vi "Configure Trigger (RS232).vi"(0 "VISA resource name":refnum<visa-resource-name>, 5 "Trigger Source (1: Bus 1)":u16(ring)=1 items=["Bus 1"=1, "Bus 2"=2, "Bus 3"=3, "Bus 4"=4], 7 "Trigger Condition (0: RX Start)":u16(ring) items=["RX Start", "RX Data", "RX End Packet", "TX Start", "TX Data", "TX End Packet"], 9 "Data":T1={"Data Size (1)"=1, "Data Value (XXXXXXXX)"="XXXXXXXX"}, 11 "error in (no error)":errorcluster) -> (4 "VISA resource name out":refnum<visa-resource-name>, 15 "error out":errorcluster)   [LabVIEW 2009, in "Tektronix DPO MSO 2000 4000 Series.lvlib"]
doc: "Configures RS232 trigger settings for the oscilloscope."
uses:
  <instrlib>/Tektronix DPO MSO 2000 4000 Series/Tektronix DPO MSO 2000 4000 Series.lvlib
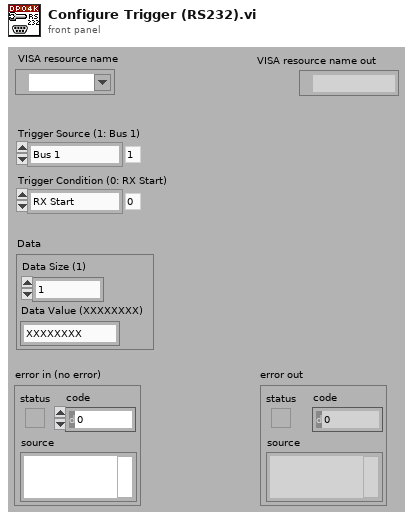
[diagram p1: front panel]
types:
  T1 = cluster{"Data Size (1)":i32, "Data Value (XXXXXXXX)":string}
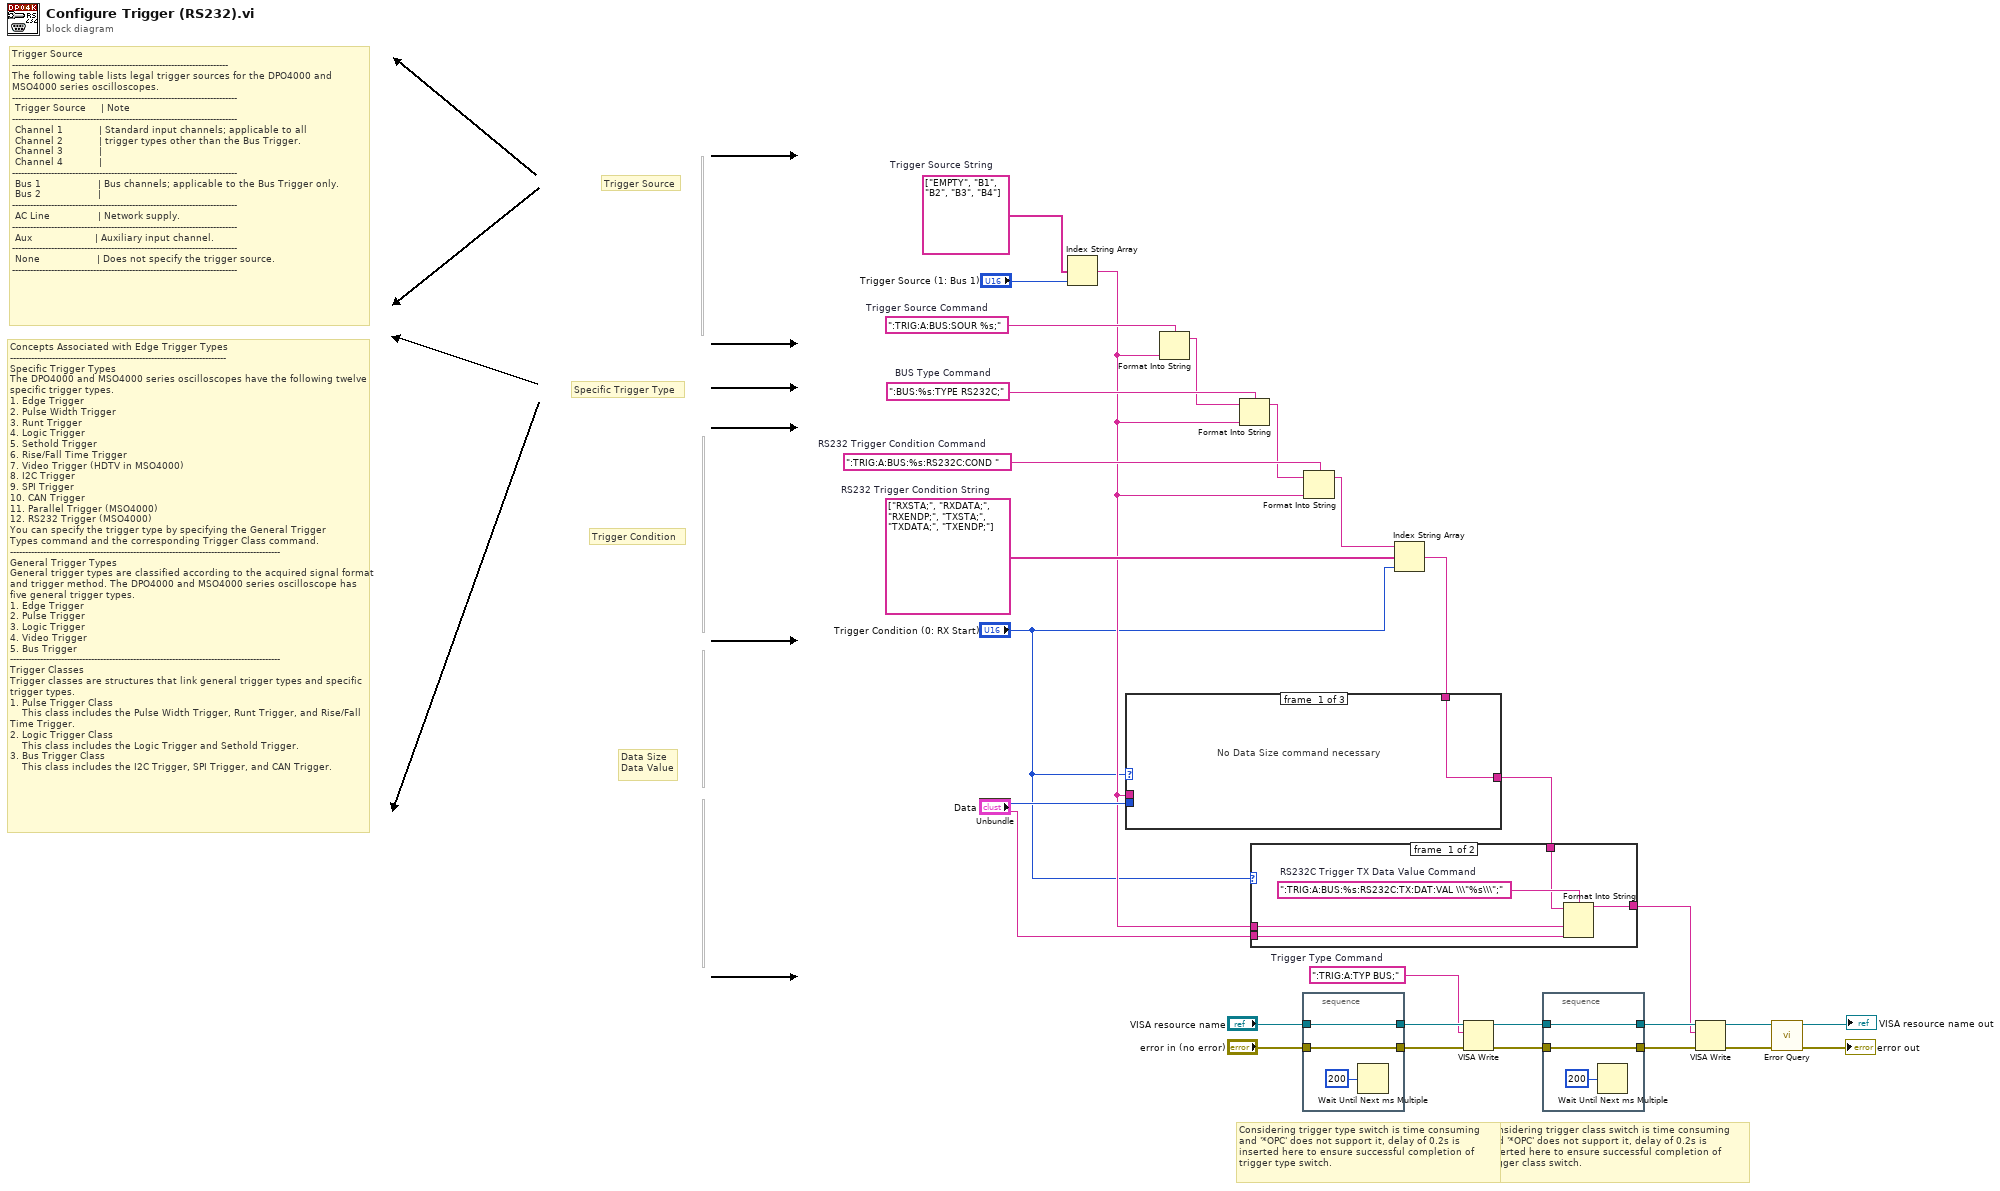
[diagram p0: block diagram]
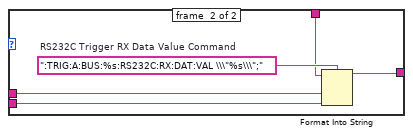
[diagram p2: hidden frame]
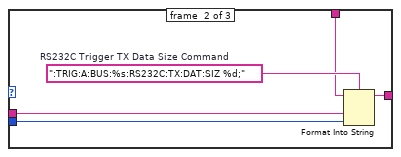
[diagram p3: hidden frame]
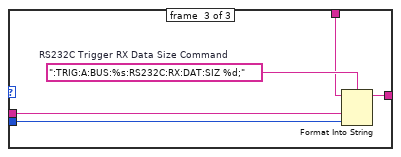
[diagram p4: hidden frame]
diagram:
  w22 = string[] ["EMPTY", "B1", "B2", "B3", "B4"]  # Trigger Source String
  w20 = ":TRIG:A:BUS:SOUR %s;"  # Trigger Source Command
  w24 = string[] ["RXSTA;", "RXDATA;", "RXENDP;", "TXSTA;", "TXDATA;", "TXENDP;"]  # RS232 Trigger Condition String
  w25 = ":TRIG:A:BUS:%s:RS232C:COND "  # RS232 Trigger Condition Command
  w21 = ":BUS:%s:TYPE RS232C;"  # BUS Type Command
  w28 = ":TRIG:A:TYP BUS;"  # Trigger Type Command
  # "Trigger Source\n------------------------------------------------------------------------\nThe following table lists legal trigger sources for the DPO4000 and MSO4000 series oscilloscopes.\n---------------------------------------------------------------------------\n Trigger Source     | Note                                                           \n---------------------------------------------------------------------------\n Channel 1            | Standard input channels; applicable to all      \n Channel 2            | trigger types other than the Bus Trigger.         \n Channel 3            |     \n Channel 4            |\n---------------------------------------------------------------------------\n Bus 1                   | Bus channels; applicable to the Bus Trigger only.\n Bus 2                   | \n---------------------------------------------------------------------------\n AC Line                | Network supply.\n---------------------------------------------------------------------------\n Aux                     | Auxiliary input channel.\n---------------------------------------------------------------------------\n None                   | Does not specify the trigger source.\n---------------------------------------------------------------------------"
  # "Concepts Associated with Edge Trigger Types\n------------------------------------------------------------------------\nSpecific Trigger Types\nThe DPO4000 and MSO4000 series oscilloscopes have the following twelve specific trigger types.\n1. Edge Trigger\n2. Pulse Width Trigger\n3. Runt Trigger\n4. Logic Trigger\n5. Sethold Trigger\n6. Rise/Fall Time Trigger\n7. Video Trigger (HDTV in MSO4000)\n8. I2C Trigger\n9. SPI Trigger\n10. CAN Trigger\n11. Parallel Trigger (MSO4000)\n12. RS232 Trigger (MSO4000)\nYou can specify the trigger type by specifying the General Trigger \nTypes command and the corresponding Trigger Class command.\n------------------------------------------------------------------------------------------\nGeneral Trigger Types \nGeneral trigger types are classified according to the acquired signal format and trigger method. The DPO4000 and MSO4000 series oscilloscope has five general trigger types.\n1. Edge Trigger\n2. Pulse Trigger\n3. Logic Trigger\n4. Video Trigger\n5. Bus Trigger\n------------------------------------------------------------------------------------------\nTrigger Classes\nTrigger classes are structures that link general trigger types and specific trigger types.\n1. Pulse Trigger Class\n    This class includes the Pulse Width Trigger, Runt Trigger, and Rise/Fall Time Trigger.\n2. Logic Trigger Class\n    This class includes the Logic Trigger and Sethold Trigger.\n3. Bus Trigger Class\n    This class includes the I2C Trigger, SPI Trigger, and CAN Trigger."
  # "Considering trigger class switch is time consuming\nand '*OPC' does not support it, delay of 0.2s is \ninserted here to ensure successful completion of\ntrigger class switch."
  # "Data Size\nData Value"
  # "Trigger Condition"
  # "Specific Trigger Type"
  # "Trigger Source"
  # "Considering trigger type switch is time consuming\nand '*OPC' does not support it, delay of 0.2s is \ninserted here to ensure successful completion of\ntrigger type switch."
  n1 = Unbundle("Data") -> ("Data Size (1)"=w8:i32, "Data Value (XXXXXXXX)"=w5:string)
  n2 = Index String Array(1:"Trigger Source (1: Bus 1)", 2:w22) -> (0:w6:string)  [unwired: 1 in]
  n3 = Format Into String(format string=w20, w6) -> (resulting string=w19:string)  [unwired: 2 in, 1 out]
  n4 = Format Into String(format string=w21, initial string=w19, w6) -> (resulting string=w18:string)  [unwired: 1 in, 1 out]
  n5 = stacked-sequence {
    tunnel: "VISA resource name" -> [w32]
    tunnel: [w32] -> w30
    tunnel: "error in (no error)" -> [w31]
    tunnel: [w31] -> w29
    frame #0 {
      n6 = Wait Until Next ms Multiple(millisecond multiple=u32 200) -> ()  [unwired: 1 out]
    }
  }
  n7 = Format Into String(format string=w25, initial string=w18, w6) -> (resulting string=w17:string)  [unwired: 1 in, 1 out]
  n8 = Index String Array(1:"Trigger Condition (0: RX Start)", 2:w24, 3:w17) -> (0:w7:string)
  n9 = case shown="0, Default" "Trigger Condition (0: RX Start)" {
    tunnel: [w34 w35 w40] -> w4
    tunnel: w6 -> [_ w36 w41]
    tunnel: w8 -> [_ w38 w43]
    tunnel: w7 -> [w34 w37 w42]
    frame #0 {
      # "No Data Size command necessary"
    }
    frame #1 {
      w39 = ":TRIG:A:BUS:%s:RS232C:TX:DAT:SIZ %d;"  # RS232C Trigger TX Data Size Command
      n10 = Format Into String(format string=w39, initial string=w37, w36, w38) -> (resulting string=w35:string)  [unwired: 1 in, 1 out]
    }
    frame #2 {
      w44 = ":TRIG:A:BUS:%s:RS232C:RX:DAT:SIZ %d;"  # RS232C Trigger RX Data Size Command
      n11 = Format Into String(format string=w44, initial string=w42, w41, w43) -> (resulting string=w40:string)  [unwired: 1 in, 1 out]
    }
  }
  n12 = case shown="0..2, Default" "Trigger Condition (0: RX Start)" {
    tunnel: [w48 w51] -> w3
    tunnel: w6 -> [w47 w54]
    tunnel: w5 -> [w46 w53]
    tunnel: w4 -> [w45 w50]
    frame #0 {
      w49 = ":TRIG:A:BUS:%s:RS232C:TX:DAT:VAL \\\"%s\\\";"  # RS232C Trigger TX Data Value Command
      n13 = Format Into String(format string=w49, initial string=w45, w47, w46) -> (resulting string=w48:string)  [unwired: 1 in, 1 out]
    }
    frame #1 {
      w52 = ":TRIG:A:BUS:%s:RS232C:RX:DAT:VAL \\\"%s\\\";"  # RS232C Trigger RX Data Value Command
      n14 = Format Into String(format string=w52, initial string=w50, w54, w53) -> (resulting string=w51:string)  [unwired: 1 in, 1 out]
    }
  }
  n15 = VISA Write(VISA resource name=w30, write buffer=w28, error in (no error)=w29) -> (VISA resource name out=w27:refnum<visa-resource-name>, error out=w26:errorcluster)  [unwired: 1 out]
  n16 = stacked-sequence {
    tunnel: w27 -> [w56]
    tunnel: [w56] -> w16
    tunnel: w26 -> [w55]
    tunnel: [w55] -> w15
    frame #0 {
      n17 = Wait Until Next ms Multiple(millisecond multiple=u32 200) -> ()  [unwired: 1 out]
    }
  }
  n18 = VISA Write(VISA resource name=w16, write buffer=w3, error in (no error)=w15) -> (VISA resource name out=w14:refnum<visa-resource-name>, error out=w13:errorcluster)  [unwired: 1 out]
  n19 = call <instrlib>:"Error Query.vi"("error in (no error)"=w13, "VISA resource name"=w14) -> ("error out"=→"error out":errorcluster, "VISA resource name out"=→"VISA resource name out":refnum<visa-resource-name>)  [unwired: 6 in, 2 out]
